vi "Simple TCP - Server.vi"(8 "error":errorcluster, 10 "ParserQueue":refnum<queue>, 11 "TCP_Queue":refnum<queue>) -> ()   [LabVIEW 2021]
doc: "Demonstrates how to set up a basic TCP connection, send data to the specified port once a connection has been established, and terminate the connection once the data has been sent. This VI is designed to stop if the TCP connection is terminated. The data sent in this example is an array of random numbers."
uses:
  Controls/Enums/Parser_Loop_Enum.ctl
  Controls/Enums/TCP_Loop_Enum.ctl
panel:
  out "Received":string
  in  "bytes to read":i32=1
  in  "Client Closed":string="The client VI closed the connection."
  in  "Stop":bool
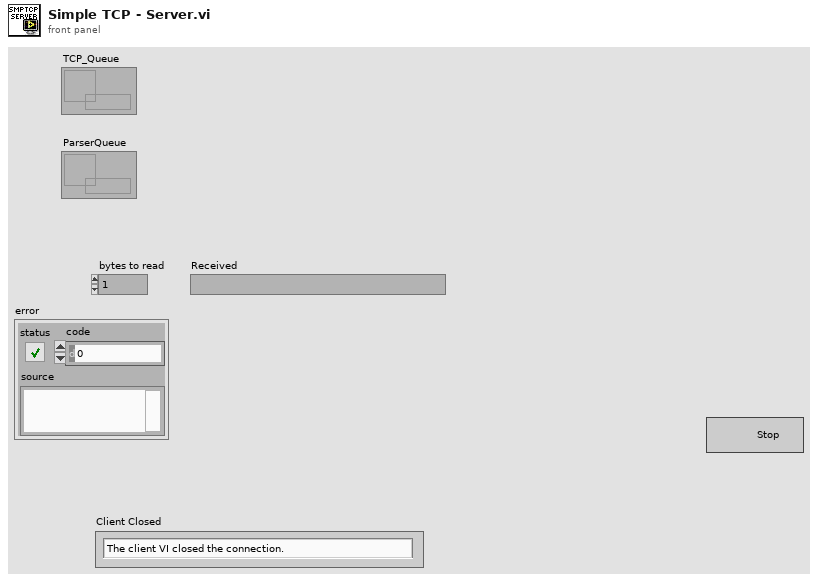
[diagram p1: front panel]
types:
  T1 = typedef "Parser_Loop_Enum.ctl" = enum16{"Init", "Receive", "Send", "Parse", "ChkTime", "Close"}
  T2 = typedef "TCP_Loop_Enum.ctl" = enum16{"TCP_Init", "TCP_Read", "TCP_Write", "TCP_Close"}
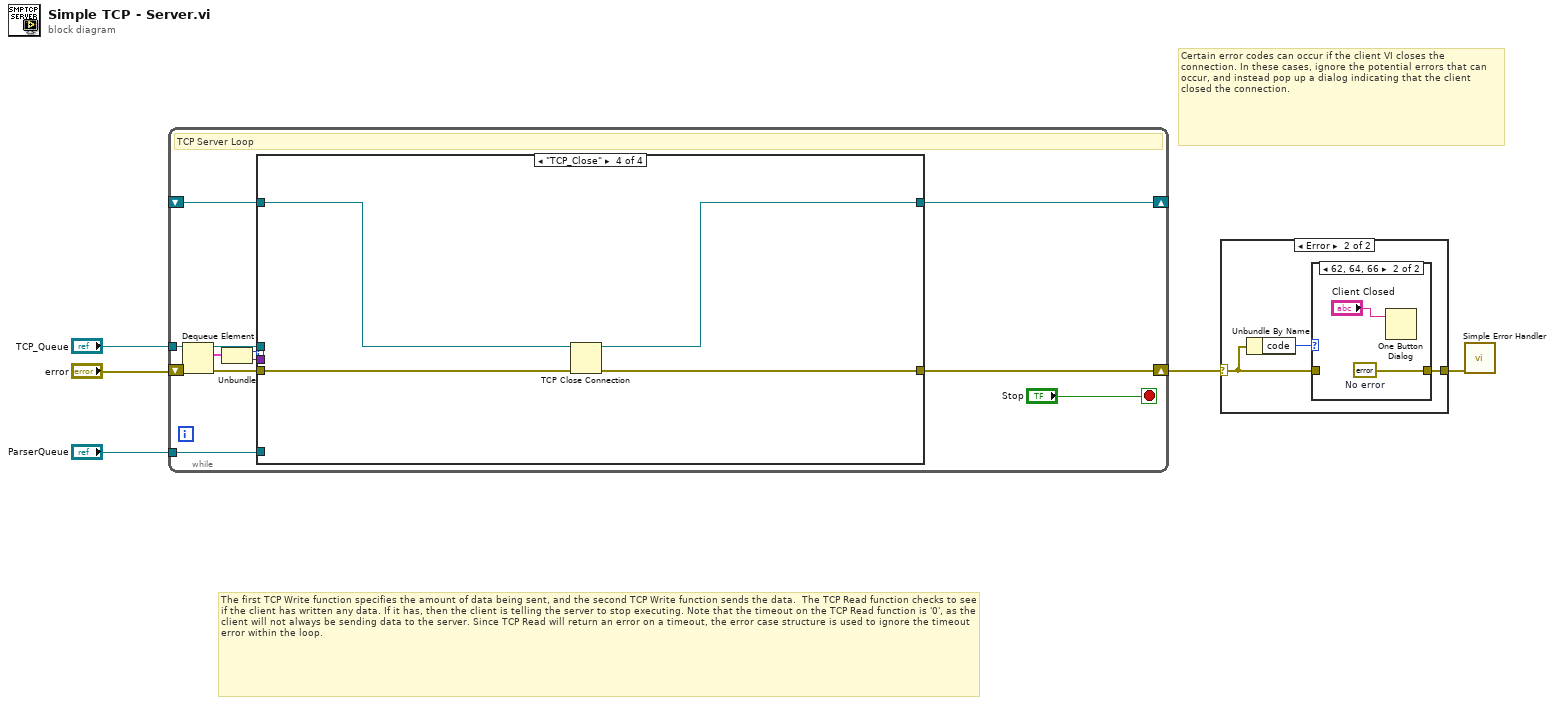
[diagram p0: block diagram]
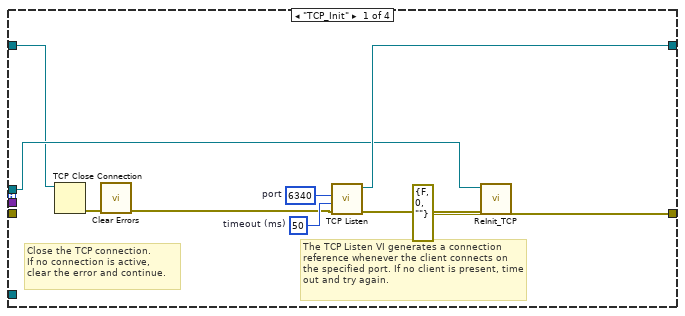
[diagram p2: hidden frame]
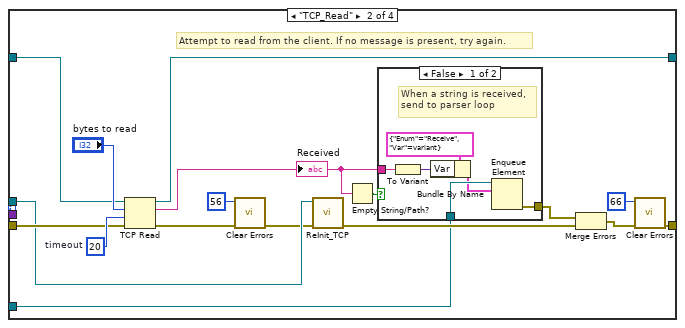
[diagram p3: hidden frame]
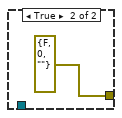
[diagram p4: hidden frame]
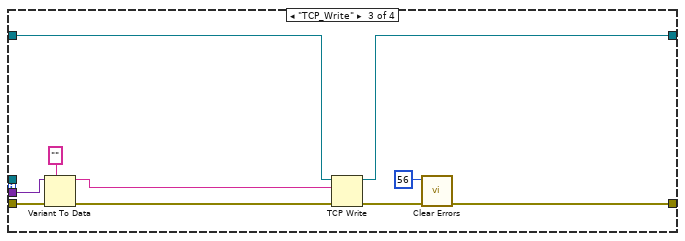
[diagram p5: hidden frame]
diagram:
  # "Certain error codes can occur if the client VI closes the connection. In these cases, ignore the potential errors that can occur, and instead pop up a dialog indicating that the client closed the connection."
  # "The first TCP Write function specifies the amount of data being sent, and the second TCP Write function sends the data.  The TCP Read function checks to see if the client has written any data. If it has, then the client is telling the server to stop executing. Note that the timeout on the TCP Read function is '0', as the client will not always be sending data to the server. Since TCP Read will return an error on a timeout, the error case structure is used to ignore the timeout error within the loop."
  n1 = while {
    shift-right: [w15] -> _
    shift-left: _ -> [w17]
    shift-right: [w14] -> w4
    shift-left: "error" -> [w13]
    tunnel: "TCP_Queue" -> [w9]
    tunnel: "ParserQueue" -> [w6]
    stop <- "Stop" stop-if-true
    # "TCP Server Loop"
    n2 = Dequeue Element(queue=w9, error in (no error)=w13) -> (queue out=w10:refnum<queue>, element=w11:cluster{T2, variant}, error out=w12:errorcluster)  [unwired: 1 in, 1 out]
    n3 = Unbundle(w11) -> (w8:T2, w7:variant)
    n4 = case shown="\"TCP_Close\"" w8 {
      tunnel: w17 -> [w20 w41 w60 w63]
      tunnel: w12 -> [_ w40 w54 w64]
      tunnel: [errorcluster {"status"=FALSE, "code"=0, "source"=""} ("error out") w28 w58 w61] -> w14
      tunnel: [w24 w36 w56 w62] -> w15
      tunnel: w10 -> [w23 w39 _ _]
      tunnel: w7 -> [_ _ w53 _]
      tunnel: w6 -> [_ w35 _ _]
      frame "TCP_Init" {
        w25 = u16 6340  # port
        w26 = 50  # timeout (ms)
        # "Close the TCP connection.\nIf no connection is active,\nclear the error and continue."
        # "The TCP Listen VI generates a connection reference whenever the client connects on the specified port. If no client is present, time out and try again."
        n5 = TCP Close Connection(connection ID=w20) -> (error out=w19:errorcluster)  [unwired: 1 in, 2 out]
        n6 = call <vilib>:"Clear Errors.vi"("error in (no error)"=w19) -> ("error out"=w18:errorcluster)  [unwired: 5 in, 1 out]
        n7 = call <vilib>:"TCP Listen.vi"("error in (no error)"=w18, "timeout ms (wait forever: -1)"=w26, "port"=w25) -> ("error out"=w22:errorcluster, "connection ID"=w24:refnum<k5>)  [unwired: 4 in, 3 out]
        n8 = call "ReInit_TCP.vi"("error in (no error)"=w22, "Queue in"=w23) -> ()  [unwired: 9 in, 1 out]
      }
      frame "TCP_Read" {
        w43 = 20  # timeout
        # "Attempt to read from the client. If no message is present, try again."
        n9 = TCP Read(connection ID=w41, bytes to read="bytes to read", error in (no error)=w40, 9:w43) -> (connection ID out=w36:refnum<k5>, data out=w32:string, error out=w38:errorcluster)  [unwired: 1 out]
        "Received" <- w32
        n10 = call <vilib>:"Clear Errors.vi"("error in (no error)"=w38, "specific error code to clear (0: all)"=56) -> ("error out"=w30:errorcluster)  [unwired: 4 in, 1 out]
        n11 = call "ReInit_TCP.vi"("error in (no error)"=w30, "Queue in"=w39) -> ("error out"=w37:errorcluster)  [unwired: 9 in]
        n12 = Empty String/Path?(string/path=w32) -> (empty?=w31:bool)
        n13 = case shown="False" w31 {
          tunnel: w35 -> [w49 _]
          tunnel: w32 -> [w45 _]
          tunnel: [w44 errorcluster {"status"=FALSE, "code"=0, "source"=""} ("error out")] -> w33
          frame False {
            # "When a string is received,\nsend to parser loop"
            n14 = To Variant(anything=w45) -> (Variant=w46:variant)
            n15 = Bundle By Name(cluster=cluster{"Enum":T1, "Var":variant} {"Enum"=enum."Receive", "Var"=variant} ("element"), "Var"=w46) -> (w47:cluster{"Enum":T1, "Var":variant})
            n16 = Enqueue Element(queue=w49, element=w47) -> (error out=w44:errorcluster)  [unwired: 2 in, 2 out]
          }
          frame True {
          }
        }
        n17 = Merge Errors(w33, w37) -> (w34:errorcluster)
        n18 = call <vilib>:"Clear Errors.vi"("error in (no error)"=w34, "specific error code to clear (0: all)"=66) -> ("error out"=w28:errorcluster)  [unwired: 4 in, 1 out]
      }
      frame "TCP_Write" {
        n19 = Variant To Data(error in=w54, type="" ("ToSend"), Variant=w53) -> (data=w51:string, error out=w55:errorcluster)
        n20 = TCP Write(connection ID=w60, data in=w51, error in (no error)=w55) -> (connection ID out=w56:refnum<k5>, error out=w59:errorcluster)  [unwired: 2 out]
        n21 = call <vilib>:"Clear Errors.vi"("error in (no error)"=w59, "specific error code to clear (0: all)"=56) -> ("error out"=w58:errorcluster)  [unwired: 4 in, 1 out]
      }
      frame "TCP_Close" {
        n22 = TCP Close Connection(connection ID=w63, error in (no error)=w64) -> (connection ID out=w62:refnum<k5>, error out=w61:errorcluster)  [unwired: 1 out]
      }
    }
  }
  n23 = case shown="Error" w4 {
    selector: w4 -> [w65 w67]
    tunnel: [w65 w66] -> w5
    frame No Error {
    }
    frame Error {
      n24 = Unbundle By Name(w67) -> ("code"=w68:i32)
      n25 = case shown="62, 64, 66" w68 {
        tunnel: w67 -> [w69 _]
        tunnel: [w69 w71] -> w66
        frame Default {
        }
        frame 62, 64, 66 {
          w71 = errorcluster {"status"=FALSE, "code"=0, "source"=""}  # No error
          n26 = One Button Dialog(message="Client Closed") -> ()  [unwired: 1 in, 1 out]
        }
      }
    }
  }
  n27 = call <vilib>:"Simple Error Handler.vi"("error in (no error)"=w5) -> ()  [unwired: 1 in, 8 out]
